vi "Destroy.vi"(8 "error in (no error)":errorcluster, 11 "dotNET Container in":refnum<class "dotNET Container.lvclass">) -> (0 "error out":errorcluster, 3 "dotNET Container out":refnum<class "dotNET Container.lvclass">)   [LabVIEW 2019, in "dotNET Container.lvclass"]
uses:
  dotNET Container.lvclass
  Container base/Container base.lvclass
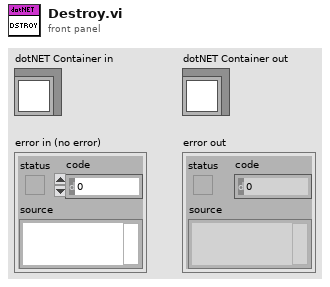
[diagram p1: front panel]
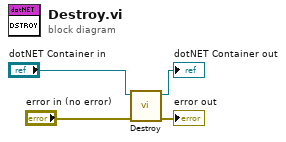
[diagram p0: block diagram]
diagram:
  n1 = call-parent "Destroy.vi"("error in (no error)"="error in (no error)", "Container base in"="dotNET Container in") -> ("error out"=→"error out":errorcluster, "Container base out"=→"dotNET Container out":refnum<class "dotNET Container.lvclass">)  [unwired: 8 in]
